vi "Helium Fridge Cool-Down.vi"() -> ()   [LabVIEW 2009]
uses:
  <vilib>/express/express signal manip/GetorSetDDTAttributes/Set DDT Attributes/Set DDT Properties.xnode
  <vilib>/express/express shared/transition.llb/Waveform Array To Dynamic.vi
  <vilib>/express/express signal manip/GetorSetDDTAttributes/Set DDT Attributes/SetT0.vi
  <vilib>/express/express shared/transition.llb/Dynamic To Waveform Array.vi
panel:
  out "Resistance Strip Chart":dynamicdata(graph)
  in  "Seconds between \nMeasurements":dbl=30.0 min=0.0 max=9999999.0 step=1.0
  out "All Clear":bool
  out "Error":bool
  out "Run Start Time":string
  out "Last Measurement Taken":string
  out "Most Recent Error":string
  out "Heartbeat":bool
  in  "Heartbeat":bool
  in  "Temp Strip Chart":bool
  out "Temperature Strip Chart":dynamicdata(graph)
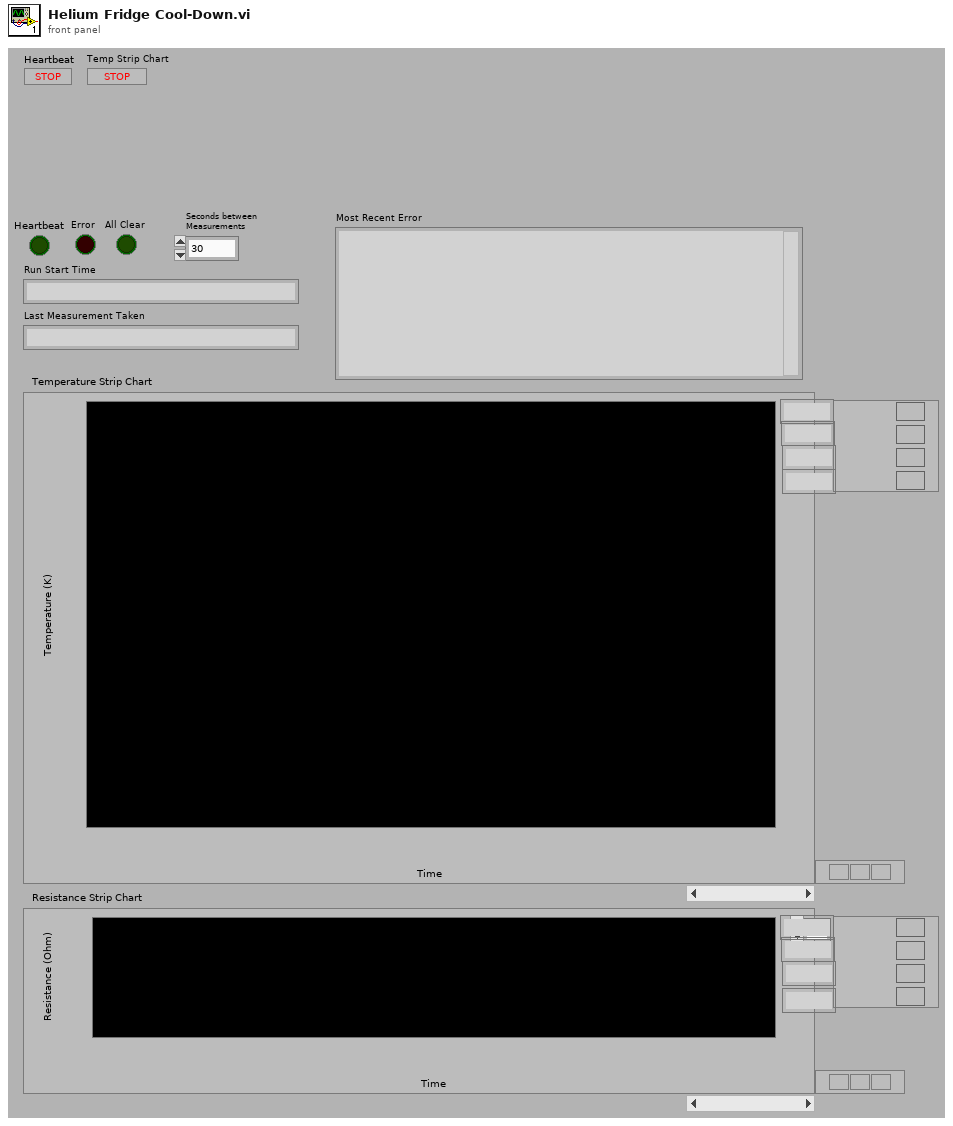
[diagram p1: front panel]
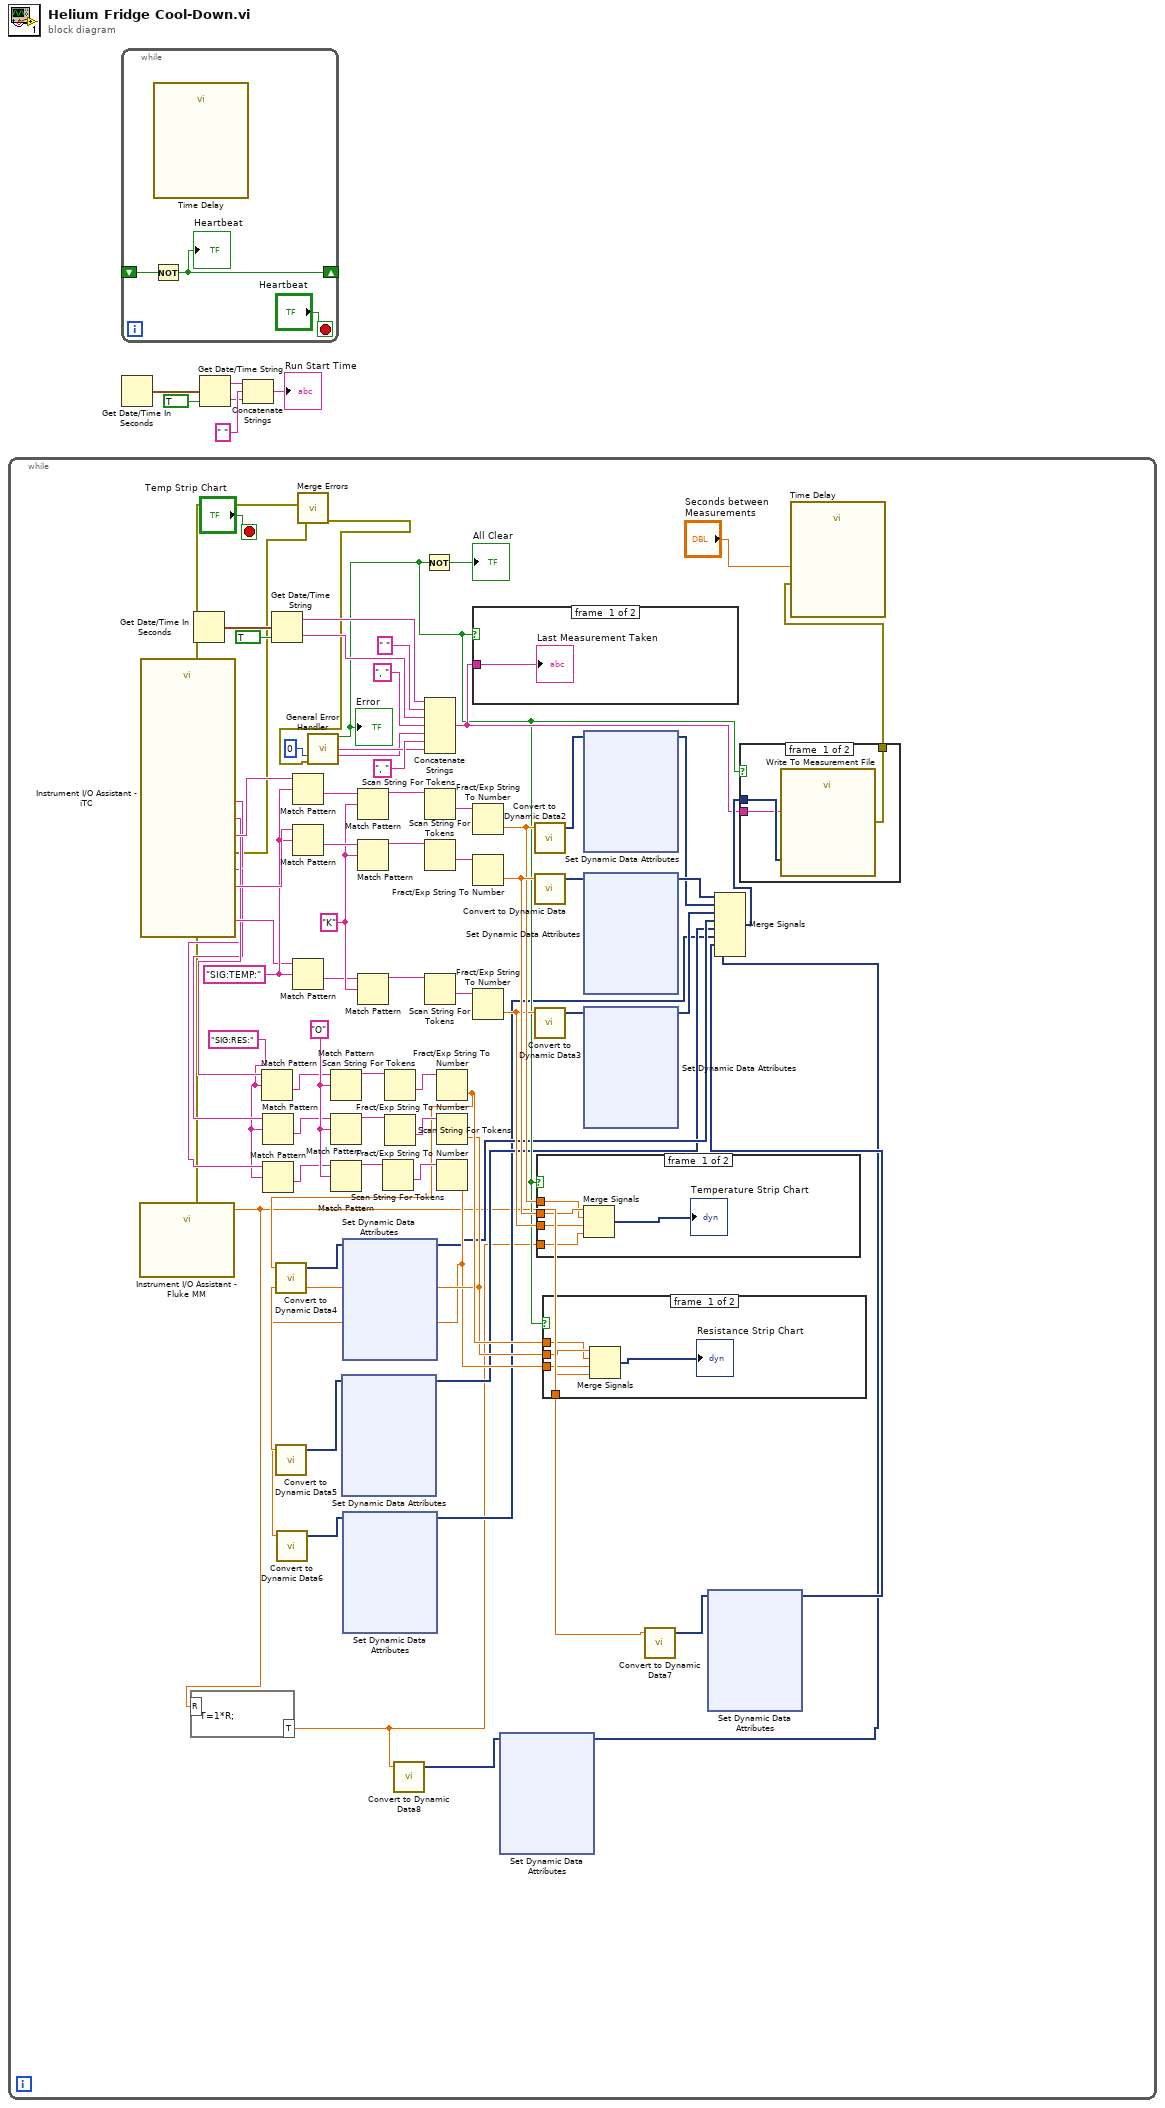
[diagram p0: block diagram]
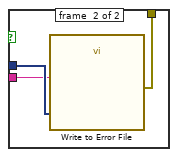
[diagram p4: hidden frame]
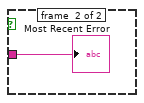
[diagram p5: hidden frame]
diagram:
  n1 = while {
    stop <- "Temp Strip Chart" stop-if-true
    w35 = "O"
    w36 = "SIG:RES:"
    w46 = "SIG:TEMP:"
    w45 = "K"
    n2 = call "Instrument I/O Assistant - Fluke MM"() -> ("AB3.R"=w10:dbl, "error out"=w11:errorcluster)  [unwired: 26 in]
    n3 = call "Instrument I/O Assistant - iTC"() -> ("AB1.R"=w37:string, "CCS.R"=w39:string, "Pill.R"=w38:string, "AB1.T"=w44:string, "CCS.T"=w49:string, "Pill.T"=w52:string, "error out"=w13:errorcluster)  [unwired: 20 in, 1 out]
    n4 = formula code="T=1*R;"("R"=w10) -> ("T"=w9:dbl)
    n5 = Get Date/Time In Seconds() -> (seconds since 1Jan1904=w74:timestamp)
    n6 = Match Pattern(string=w39, regular expression=w36) -> (after substring=w34:string)  [unwired: 1 in, 3 out]
    n7 = Match Pattern(string=w38, regular expression=w36) -> (after substring=w33:string)  [unwired: 1 in, 3 out]
    n8 = Match Pattern(string=w37, regular expression=w36) -> (after substring=w32:string)  [unwired: 1 in, 3 out]
    n9 = Get Date/Time String(seconds (now)=w74, want seconds? (F)=TRUE) -> (date string=w72:string, time string=w70:string)  [unwired: 1 in]
    n10 = Match Pattern(string=w49, regular expression=w46) -> (after substring=w48:string)  [unwired: 1 in, 3 out]
    n11 = Match Pattern(string=w52, regular expression=w46) -> (after substring=w51:string)  [unwired: 1 in, 3 out]
    n12 = Match Pattern(string=w44, regular expression=w46) -> (after substring=w43:string)  [unwired: 1 in, 3 out]
    n13 = call <vilib>:"Merge Errors.vi"("error in 2 (no error)"=w11, "error in 1 (no error)"=w13) -> ("error out"=w12:errorcluster)  [unwired: 5 in]
    n14 = call <vilib>:"General Error Handler.vi"("type of dialog (OK msg:1)"=0, "error in (no error)"=w12) -> ("error?"=w25:bool, "source out"=w58:string, "message"=w57:string)  [unwired: 9 in, 2 out]
    "Error" <- w25
    n15 = Match Pattern(string=w34, regular expression=w35) -> (before substring=w31:string)  [unwired: 1 in, 3 out]
    n16 = Match Pattern(string=w33, regular expression=w35) -> (before substring=w30:string)  [unwired: 1 in, 3 out]
    n17 = Match Pattern(string=w32, regular expression=w35) -> (before substring=w29:string)  [unwired: 1 in, 3 out]
    n18 = Match Pattern(string=w48, regular expression=w45) -> (before substring=w47:string)  [unwired: 1 in, 3 out]
    n19 = Match Pattern(string=w51, regular expression=w45) -> (before substring=w50:string)  [unwired: 1 in, 3 out]
    n20 = Match Pattern(string=w43, regular expression=w45) -> (before substring=w42:string)  [unwired: 1 in, 3 out]
    n21 = Scan String For Tokens(9:w29) -> (1:w26:string)  [unwired: 5 in, 3 out]
    n22 = Scan String For Tokens(9:w31) -> (1:w28:string)  [unwired: 5 in, 3 out]
    n23 = Scan String For Tokens(9:w30) -> (1:w27:string)  [unwired: 5 in, 3 out]
    n24 = call "Convert to Dynamic Data8"("Double"=w9) -> ("Dynamic Data Type"=w8:dynamicdata)  [unwired: 3 in]
    n25 = Not(x=w25) -> (.not. x?=→"All Clear":bool)
    n26 = Concatenate Strings(w72, " ", w70, ", ", w57, ", ", w58) -> (w55:string)
    n27 = Scan String For Tokens(9:w47) -> (1:w76:string)  [unwired: 5 in, 3 out]
    n28 = Scan String For Tokens(9:w50) -> (1:w78:string)  [unwired: 5 in, 3 out]
    n29 = Scan String For Tokens(9:w42) -> (1:w75:string)  [unwired: 5 in, 3 out]
    n30 = Fract/Exp String To Number(string=w28) -> (number=w24:dbl)  [unwired: 3 in, 1 out]
    n31 = call "Convert to Dynamic Data4"("Double"=w24) -> ("Dynamic Data Type"=w21:dynamicdata)  [unwired: 3 in]
    n32 = xnode "Set Dynamic Data Attributes"("Signals In"=w21) -> ("Signals Out"=w18:dynamicdata)  [unwired: 4 in, 1 out]
    n33 = Fract/Exp String To Number(string=w27) -> (number=w23:dbl)  [unwired: 3 in, 1 out]
    n34 = call "Convert to Dynamic Data5"("Double"=w23) -> ("Dynamic Data Type"=w20:dynamicdata)  [unwired: 3 in]
    n35 = xnode "Set Dynamic Data Attributes"("Signals In"=w20) -> ("Signals Out"=w17:dynamicdata)  [unwired: 4 in, 1 out]
    n36 = Fract/Exp String To Number(string=w26) -> (number=w22:dbl)  [unwired: 3 in, 1 out]
    n37 = call "Convert to Dynamic Data6"("Double"=w22) -> ("Dynamic Data Type"=w19:dynamicdata)  [unwired: 3 in]
    n38 = xnode "Set Dynamic Data Attributes"("Signals In"=w19) -> ("Signals Out"=w16:dynamicdata)  [unwired: 4 in, 1 out]
    n39 = case shown="False" w25 {
      tunnel: w55 -> [w239 w240]
      frame #0 {
        "Last Measurement Taken" <- w239
      }
      frame #1 {
        "Most Recent Error" <- w240
      }
    }
    n40 = Fract/Exp String To Number(string=w76) -> (number=w60:dbl)  [unwired: 3 in, 1 out]
    n41 = Fract/Exp String To Number(string=w78) -> (number=w61:dbl)  [unwired: 3 in, 1 out]
    n42 = Fract/Exp String To Number(string=w75) -> (number=w59:dbl)  [unwired: 3 in, 1 out]
    n43 = xnode "Set Dynamic Data Attributes"("Signals In"=w8) -> ("Signals Out"=w7:dynamicdata)  [unwired: 4 in, 1 out]
    n44 = call "Convert to Dynamic Data2"("Double"=w60) -> ("Dynamic Data Type"=w65:dynamicdata)  [unwired: 3 in]
    n45 = call "Convert to Dynamic Data"("Double"=w61) -> ("Dynamic Data Type"=w67:dynamicdata)  [unwired: 3 in]
    n46 = call "Convert to Dynamic Data3"("Double"=w59) -> ("Dynamic Data Type"=w64:dynamicdata)  [unwired: 3 in]
    n47 = case shown="False" w25 {
      tunnel: w61 -> [w177 _]
      tunnel: w60 -> [w176 _]
      tunnel: w59 -> [w175 _]
      tunnel: w9 -> [w174 _]
      frame #0 {
        n48 = Merge Signals(w177, w176, w175, w174) -> (→"Temperature Strip Chart":dynamicdata)
      }
      frame #1 {
      }
    }
    n49 = case shown="False" w25 {
      tunnel: w23 -> [w172 _]
      tunnel: w24 -> [w171 _]
      tunnel: w22 -> [w170 _]
      tunnel: w10 -> [w169 _]
      frame #0 {
        n50 = Merge Signals(w172, w171, w170, w169) -> (→"Resistance Strip Chart":dynamicdata)
      }
      frame #1 {
      }
    }
    n51 = xnode "Set Dynamic Data Attributes"("Signals In"=w65) -> ("Signals Out"=w63:dynamicdata)  [unwired: 4 in, 1 out]
    n52 = xnode "Set Dynamic Data Attributes"("Signals In"=w67) -> ("Signals Out"=w66:dynamicdata)  [unwired: 4 in, 1 out]
    n53 = xnode "Set Dynamic Data Attributes"("Signals In"=w64) -> ("Signals Out"=w62:dynamicdata)  [unwired: 4 in, 1 out]
    n54 = call "Convert to Dynamic Data7"("Double"=w10) -> ("Dynamic Data Type"=w15:dynamicdata)  [unwired: 3 in]
    n55 = xnode "Set Dynamic Data Attributes"("Signals In"=w15) -> ("Signals Out"=w14:dynamicdata)  [unwired: 4 in, 1 out]
    n56 = Merge Signals(w66, w63, w62, w18, w17, w16, w14, w7) -> (w56:dynamicdata)
    n57 = case shown="True" w25 {
      tunnel: w56 -> [w181 w184]
      tunnel: w55 -> [w180 w183]
      tunnel: [w179 w182] -> w41
      frame #0 {
        n58 = call "Write To Measurement File"("Signals"=w181, "Comment"=w180) -> ("error out"=w179:errorcluster)  [unwired: 15 in, 2 out]
      }
      frame #1 {
        n59 = call "Write to Error File"("Signals"=w184, "Comment"=w183) -> ("error out"=w182:errorcluster)  [unwired: 15 in, 2 out]
      }
    }
    n60 = call "Time Delay"("error in (no error)"=w41, "Delay Time (s)"="Seconds between \nMeasurements") -> ()  [unwired: 9 in, 1 out]
  }
  n61 = while {
    shift-right: [w241] -> _
    shift-left: _ -> [w243]
    stop <- "Heartbeat" stop-if-true
    n62 = Not(x=w243) -> (.not. x?=w241:bool)
    "Heartbeat" <- w241
    n63 = call "Time Delay"() -> ()  [unwired: 11 in, 1 out]
  }
  n64 = Get Date/Time In Seconds() -> (seconds since 1Jan1904=w5:timestamp)
  n65 = Get Date/Time String(seconds (now)=w5, want seconds? (F)=TRUE) -> (date string=w4:string, time string=w2:string)  [unwired: 1 in]
  n66 = Concatenate Strings(w4, " ", w2) -> (→"Run Start Time":string)
